vi "DAQ setup_2.vi"(0 "Vx_min":dbl, 1 "Vx_max":dbl, 2 "数组":waveform(dbl)[](array[waveform]), 5 "rate":dbl, 7 "physical channels write":tag, 9 "Timing source":tag, 12 "sample mode":i32, 13 "physical channels read":tag, 14 "Number of samples per channel":i32) -> (4 "Writing task out":refnum<k21>, 6 "Reading task out":refnum<k21>, 15 "错误输出":errorcluster)   [LabVIEW 2013]
uses:
  <vilib>/DAQmx/write.llb/DAQmx Write (Analog 1D Wfm NChan NSamp).vi
  <vilib>/DAQmx/create/channels.llb/DAQmx Create Channel (AI-Voltage-Basic).vi
  <vilib>/DAQmx/configure/timing.llb/DAQmx Timing (Sample Clock).vi
  <vilib>/DAQmx/create/channels.llb/DAQmx Create Channel (AO-Voltage-Basic).vi
  <vilib>/DAQmx/configure/trigger.llb/DAQmx Start Trigger (Digital Edge).vi
  <vilib>/DAQmx/miscellaneous.llb/DAQmx Fill In Error Info.vi
  <resource>/objmgr/daqmx.rc
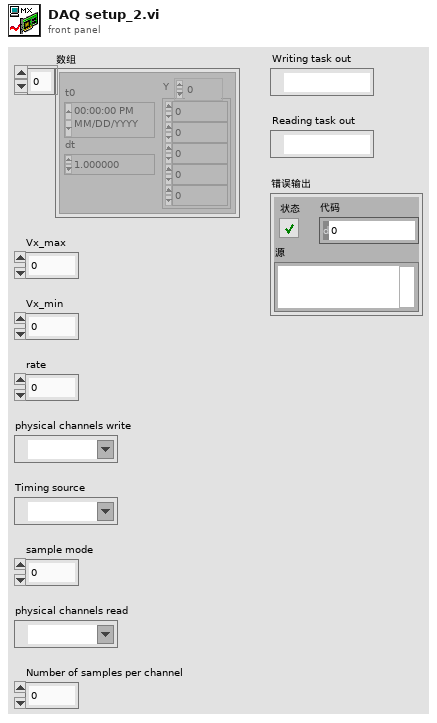
[diagram p1: front panel]
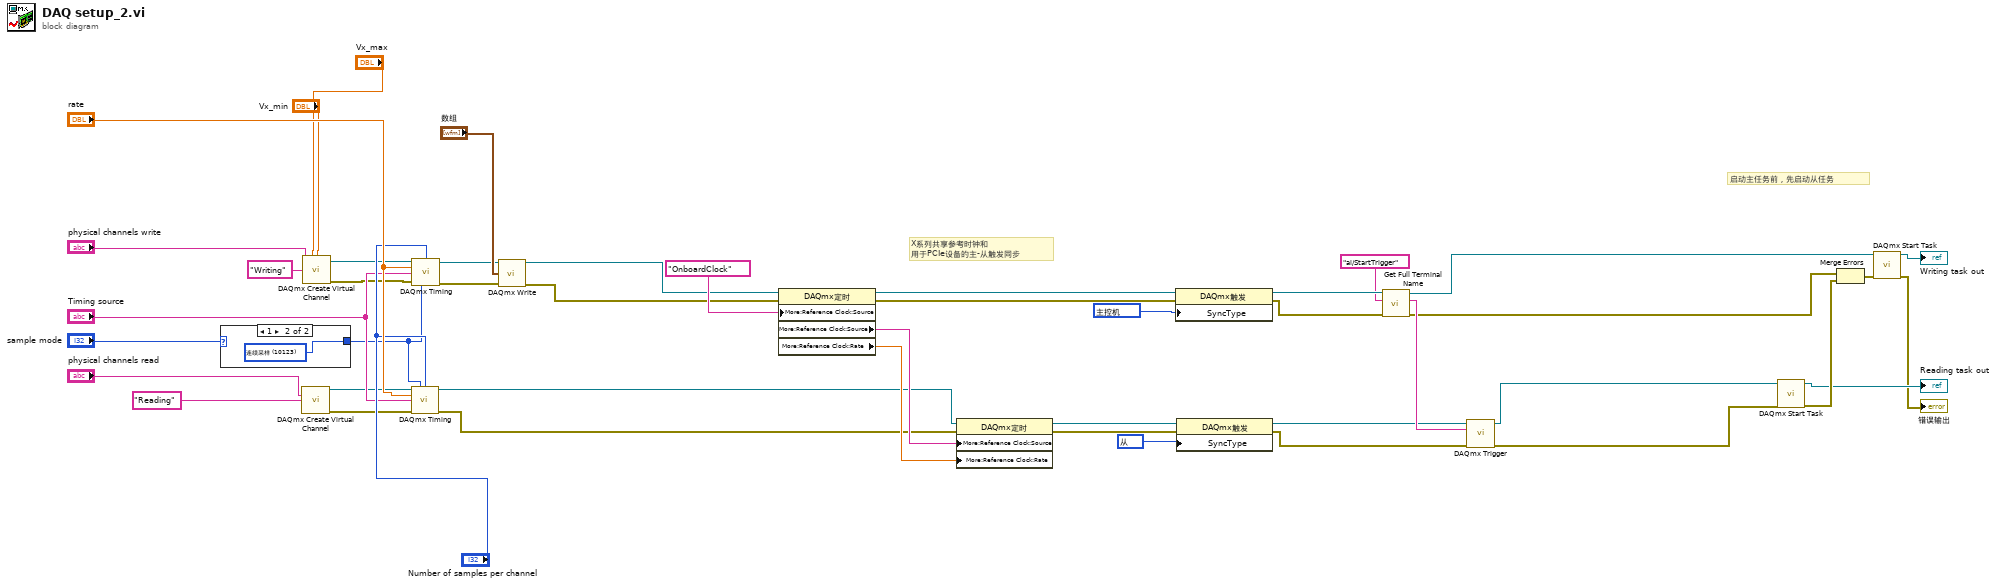
[diagram p0: block diagram]
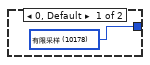
[diagram p2: hidden frame]
diagram:
  w20 = 15889 items=["无"=10230, "主控机"=15888, "从"=15889] ("同步类型")
  w21 = 15888 items=["无"=10230, "主控机"=15888, "从"=15889] ("同步类型")
  # "启动主任务前，先启动从任务"
  # "X系列共享参考时钟和\n用于PCIe设备的主-从触发同步"
  n1 = case shown="1" "sample mode" {
    tunnel: [w47 w48] -> w30
    frame 0, Default {
      w47 = 10178 items=["有限采样"=10178, "连续采样"=10123, "硬件定时单点"=12522] ("sample mode")
    }
    frame 1 {
      w48 = 10123 items=["有限采样"=10178, "连续采样"=10123, "硬件定时单点"=12522] ("sample mode")
    }
  }
  n2 = call-poly <vilib>:"DAQmx Create Virtual Channel.vi"("physical channels"="physical channels read", "name to assign"="Reading") -> ("task out"=w32:refnum<k21>, "error out"=w33:errorcluster)  [unwired: 12 in]
  n3 = call-poly <vilib>:"DAQmx Create Virtual Channel.vi"("maximum value"="Vx_max", "minimum value"="Vx_min", "physical channels"="physical channels write", "name to assign"="Writing") -> ("task out"=w36:refnum<k21>, "error out"=w37:errorcluster)  [unwired: 10 in]
  n4 = call-poly <vilib>:"DAQmx Timing.vi"("task/channels in"=w32, "sample mode"=w30, "samples per channel"="Number of samples per channel", "rate"="rate", "source"="Timing source", "error in"=w33) -> ("task out"=w17:refnum<k21>, "error out"=w16:errorcluster)  [unwired: 8 in]
  n5 = call-poly <vilib>:"DAQmx Timing.vi"("task/channels in"=w36, "sample mode"=w30, "samples per channel"="Number of samples per channel", "rate"="rate", "source"="Timing source", "error in"=w37) -> ("task out"=w34:refnum<k21>, "error out"=w35:errorcluster)  [unwired: 8 in]
  n6 = call-poly <vilib>:"DAQmx Write.vi"("task/channels in"=w34, "data"="数组", "error in"=w35) -> ("task out"=w19:refnum<k21>, "error out"=w18:errorcluster)  [unwired: 10 in, 1 out]
  n7 = property class="DAQmx定时"(reference=w19, error in=w18, "More:Reference Clock:Source"=tag "OnboardClock" ("参考时钟.源")) -> (reference out=w23:refnum<k21>, error out=w22:errorcluster, "More:Reference Clock:Source"=w28:tag, "More:Reference Clock:Rate"=w27:dbl)
  n8 = property class="DAQmx定时"(reference=w17, error in=w16, "More:Reference Clock:Source"=w28, "More:Reference Clock:Rate"=w27) -> (reference out=w25:refnum<k21>, error out=w24:errorcluster)
  n9 = property class="DAQmx触发"(reference=w23, error in=w22, "SyncType"=w21) -> (reference out=w14:refnum<k21>, error out=w13:errorcluster)
  n10 = property class="DAQmx触发"(reference=w25, error in=w24, "SyncType"=w20) -> (reference out=w11:refnum<k21>, error out=w10:errorcluster)
  n11 = call "Get Full Terminal Name.vi"("错误输入"=w13, "本地接线端名"="ai/StartTrigger", "任务/通道输入"=w14) -> ("错误输出"=w7:cluster{"状态":bool, "代码":i32, "源":string}, "带设备前缀的接线端名"=w15:tag, "任务输出"=w8:refnum<k21>)  [unwired: 6 in]
  n12 = call-poly <vilib>:"DAQmx Trigger.vi"("task/channels in"=w11, "source"=w15, "error in"=w10) -> ("task out"=w2:refnum<k21>, "error out"=w1:errorcluster)  [unwired: 11 in]
  n13 = call <vilib>:"DAQmx Start Task.vi"("task/channels in"=w2, "error in"=w1) -> ("task out"=→"Reading task out":refnum<k21>, "error out"=w6:errorcluster)  [unwired: 12 in]
  n14 = Merge Errors(w7, w6) -> (w9:errorcluster)
  n15 = call <vilib>:"DAQmx Start Task.vi"("task/channels in"=w8, "error in"=w9) -> ("task out"=→"Writing task out":refnum<k21>, "error out"=→"错误输出":errorcluster)  [unwired: 12 in]
